vi "AppendLayout_StringsAndValues.vi"(9 "StringsAndValues[] to apend":T1, 10 "SetList Layout Ref":refnum<vi>) -> ()   [LabVIEW 2013]
doc: "Append user layouts to existing layout ring StringsAndValues[]."
uses:
  <vilib>/Utility/miscctls.llb/LVStringsAndValuesArrayTypeDef_I32.ctl
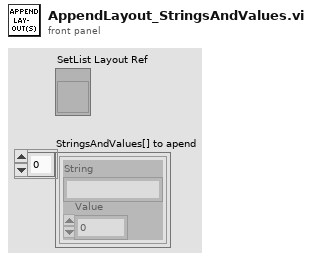
[diagram p1: front panel]
types:
  T1 = typedef "LVStringsAndValuesArrayTypeDef_I32.ctl" = cluster{"String":string, "Value":i32}[]
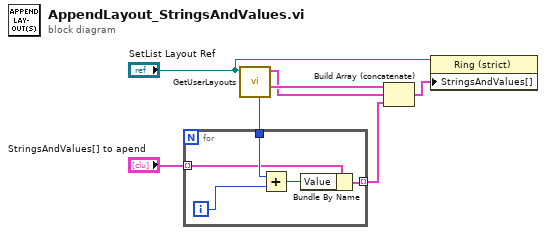
[diagram p0: block diagram]
diagram:
  n1 = call "GetUserLayouts.vi"("Layout Ring Refnum"="SetList Layout Ref") -> ("Non-user Strings And Values []"=w5:T1, "User StringsAndValues[]"=w4:T1, "Num User Layouts"=w7:i32)  [unwired: 6 in, 2 out]
  n2 = for {
    tunnel: w7 -> [w12]
    tunnel: "StringsAndValues[] to apend" -> [w11] mode=indexing
    tunnel: [w9] -> w3 mode=indexing
    i -> [w8]
    n3 = Add(x=w12, y=w8) -> (x+y=w10:i32)
    n4 = Bundle By Name(cluster=w11, "Value"=w10) -> (w9:cluster{"String":string, "Value":i32})
  }
  n5 = Build Array (concatenate)(w5, w4, w3) -> (w1:T1)
  n6 = property class="Ring (strict)"(reference="SetList Layout Ref", "StringsAndValues[]"=w1) -> ()  [unwired: 1 in, 2 out]
